vi "DC_res.vi"(1 "read buffer in":string) -> (0 "read buffer out":string)   [LabVIEW 2016]
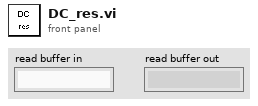
[diagram p1: front panel]
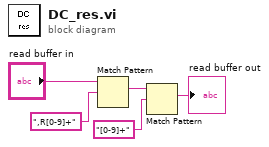
[diagram p0: block diagram]
diagram:
  n1 = Match Pattern(string="read buffer in", regular expression=",R[0-9]+") -> (match substring=w3:string)  [unwired: 1 in, 3 out]
  n2 = Match Pattern(string=w3, regular expression="[0-9]+") -> (match substring=→"read buffer out":string)  [unwired: 1 in, 3 out]
